vi "4155C Config Display.vi"(4 "Ymax":dbl format="%.2e", 5 "Var1 Stop":dbl format="%.2f", 6 "Ymin":dbl format="%.2e", 7 "Var1 Start":dbl format="%.2f", 8 "error in (no error)":errorcluster, 9 "Logarithmic":bool=TRUE, 10 "SPA Display":bool, 11 "VISA session":refnum<visa-resource-name>) -> (0 "error out":errorcluster, 3 "dup VISA resource name":refnum<visa-resource-name>)   [LabVIEW 2016]
doc: "This VI configures the timing parameters of the measurement functions. The settings of this VI could be different from the actual instrument's settings due to limits imposed by other parameters inside the instrument. To check the actual values of integration time and number of power line cycles, run HP415xA Query Integration Time.vi."
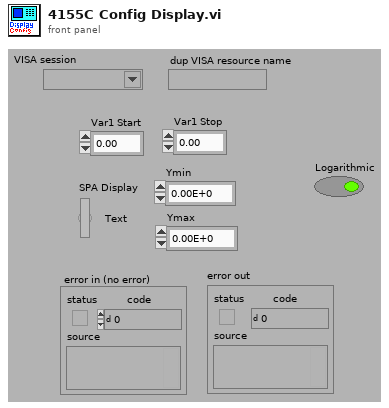
[diagram p1: front panel]
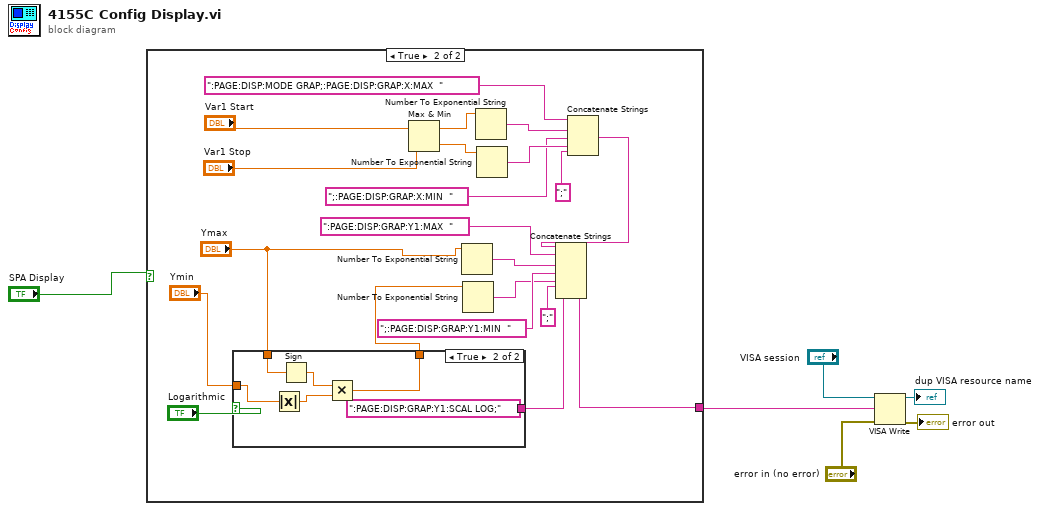
[diagram p0: block diagram]
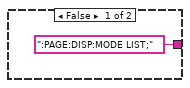
[diagram p2: hidden frame]
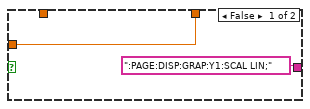
[diagram p3: hidden frame]
diagram:
  n1 = case shown="True" "SPA Display" {
    tunnel: [":PAGE:DISP:MODE LIST;" w13] -> w4
    frame False {
    }
    frame True {
      n2 = case shown="True" "Logarithmic" {
        tunnel: [":PAGE:DISP:GRAP:Y1:SCAL LIN;" ":PAGE:DISP:GRAP:Y1:SCAL LOG;"] -> w14
        tunnel: "Ymax" -> [_ w33]
        tunnel: "Ymin" -> [w29 w32]
        tunnel: [w29 w31] -> w8
        frame False {
        }
        frame True {
          n3 = Absolute Value(x=w32) -> (abs(x)=w35:dbl)
          n4 = Sign(1:w33) -> (0:w34:dbl)
          n5 = Multiply(x=w34, y=w35) -> (x*y=w31:dbl)
        }
      }
      n6 = Max & Min(x="Var1 Start", y="Var1 Stop") -> (max(x,y)=w28:dbl, min(x,y)=w27:dbl)
      n7 = Number To Exponential String(number="Ymax") -> (E-format string=w18:string)  [unwired: 3 in]
      n8 = Number To Exponential String(number=w8) -> (E-format string=w17:string)  [unwired: 3 in]
      n9 = Number To Exponential String(number=w28) -> (E-format string=w25:string)  [unwired: 3 in]
      n10 = Number To Exponential String(number=w27) -> (E-format string=w26:string)  [unwired: 3 in]
      n11 = Concatenate Strings(":PAGE:DISP:MODE GRAP;:PAGE:DISP:GRAP:X:MAX  " ("write buffer (\"\")"), w25, ";:PAGE:DISP:GRAP:X:MIN  " ("write buffer (\"\")"), w26, ";" ("Substring")) -> (w16:string)
      n12 = Concatenate Strings(w16, ":PAGE:DISP:GRAP:Y1:MAX  " ("write buffer (\"\")"), w18, ";:PAGE:DISP:GRAP:Y1:MIN  " ("write buffer (\"\")"), w17, ";" ("Substring"), w14) -> (w13:string)
    }
  }
  n13 = VISA Write(VISA resource name="VISA session", write buffer=w4, error in (no error)="error in (no error)") -> (VISA resource name out=→"dup VISA resource name":refnum<visa-resource-name>, error out=→"error out":errorcluster)  [unwired: 1 out]
